vi "编码输出.vi"(8 "error in (no error)":errorcluster, 11 "SingleStepTestV3输入":refnum<class "SingleStepCODMnV2.lvclass">) -> (0 "error out":errorcluster)   [LabVIEW 2016, in "SingleStepCODMnV2.lvlib" / "SingleStepCODMnV2.lvclass"]
uses:
  SingleStepCODMnV2.lvclass
  SingleStepCODMnV2.lvclass/SingleStepCODMnV2.ctl
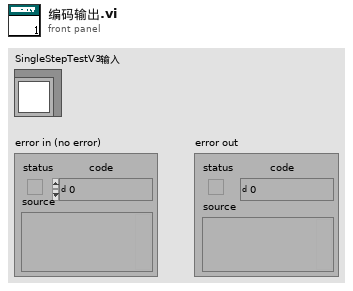
[diagram p1: front panel]
types:
  T1 = enum32{"未选择", "水样", "纯水", "标液", "零点", "加标回收", "加标回收 2"}
  T2 = enum32{"未选择", "纯水-进", "纯水-排", "硫酸-进", "硫酸-排", "复位", "高锰酸钾-进", "高锰酸钾-排", "草酸钠-进", "草酸钠-排", "氢氧化钠-进", "氢氧化钠-排", "反滴定"}
  T3 = enum32{"未选择", "V1", "V2", "V3", "V4", "V5", "V6", "V7", "V8", "V9", "V10", "V11", "V12"}
  T4 = typedef "SingleStepCODMnV2.lvlib/SingleStepCODMnV2.lvclass/State Data.ctl" = cluster{"data":u16[], "模式选择":enum16{"测试模式", "流程模式"}}
  T5 = enum32{"未选择", "水样", "纯水", "标液", "零点", "加标回收", "跨度"}
  T6 = cluster{"排液":bool, "搅拌":bool, "风扇":bool, "废液分离":bool}
  T7 = cluster{"排液阀":bool, "搅拌":bool, "冷凝风扇":bool, "废液分离阀":bool, "电磁阀1":bool, "电磁阀2":bool, "电磁阀3":bool, "电磁阀4":bool, "电磁阀5":bool, "电磁阀6":bool, "电磁阀7":bool}
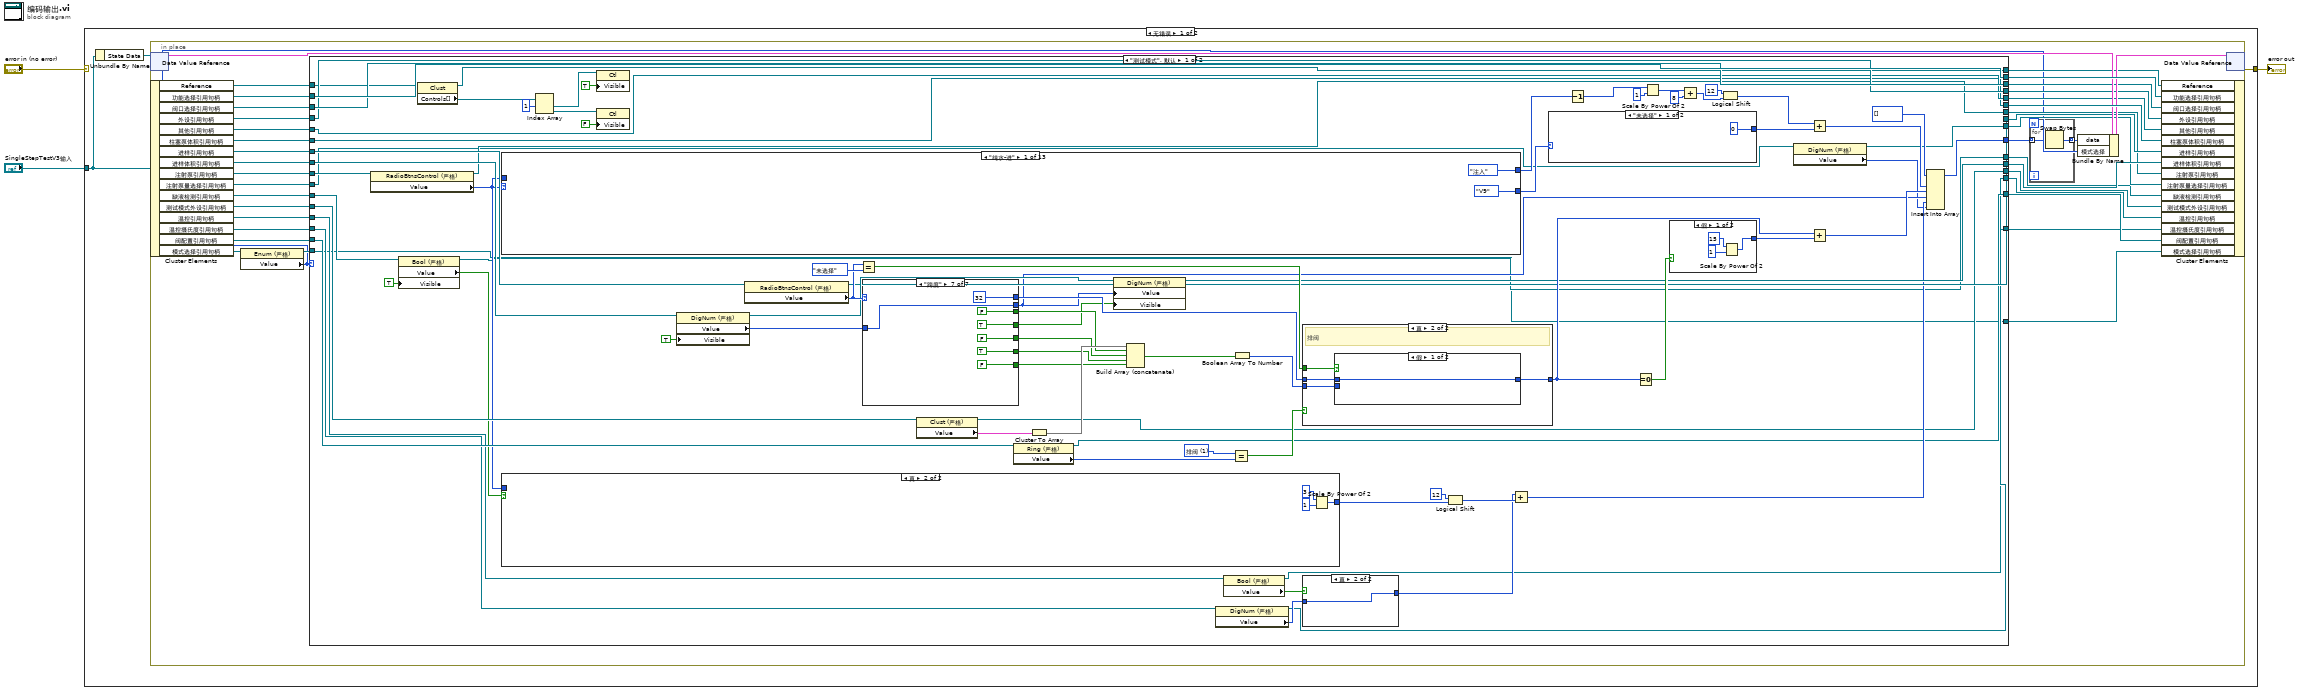
[diagram p0: block diagram]
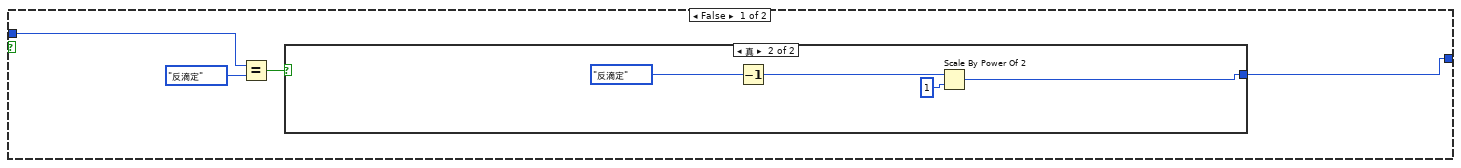
[diagram p2: hidden frame]
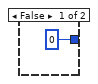
[diagram p3: hidden frame]
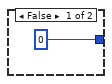
[diagram p4: hidden frame]
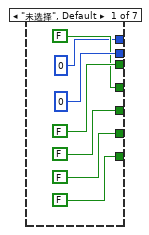
[diagram p5: hidden frame]
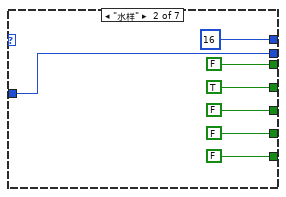
[diagram p6: hidden frame]
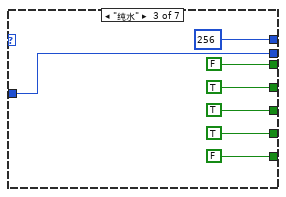
[diagram p7: hidden frame]
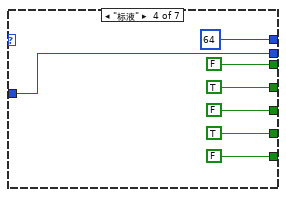
[diagram p8: hidden frame]
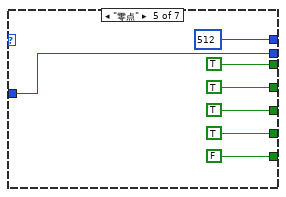
[diagram p9: hidden frame]
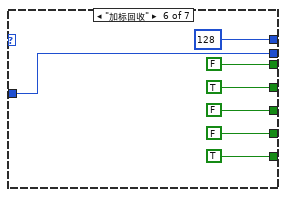
[diagram p10: hidden frame]
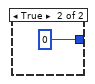
[diagram p13: hidden frame]
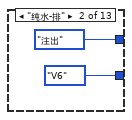
[diagram p14: hidden frame]
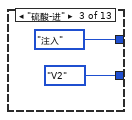
[diagram p15: hidden frame]
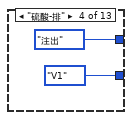
[diagram p16: hidden frame]
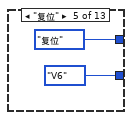
[diagram p17: hidden frame]
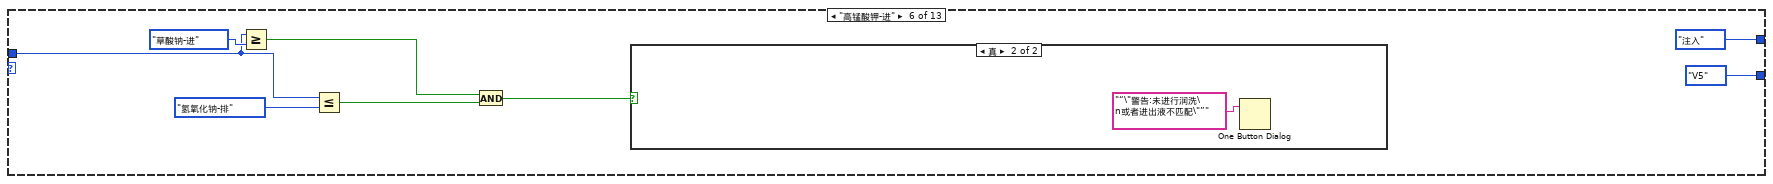
[diagram p18: hidden frame]
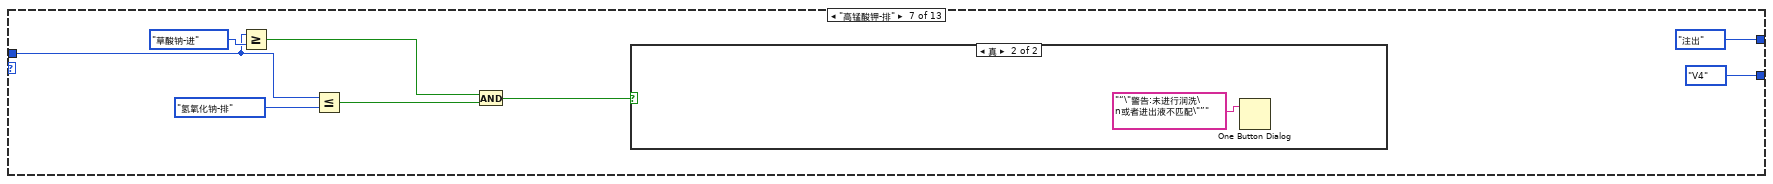
[diagram p20: hidden frame]
diagram:
  n1 = case shown="无错误" "error in (no error)" {
    selector: "error in (no error)" -> [_ w360]
    tunnel: "SingleStepTestV3输入" -> [w5 _]
    tunnel: [w4 w360] -> w2
    frame No Error {
      n2 = Unbundle By Name(w5) -> ("State Data"=w6:refnum<data-value>)
      n3 = in-place {
        n4 = in-place-dvr #1(w6) -> (w40:T4)  [unwired: 1 out]
        n5 = in-place-cluster #2(w5) -> ("Reference"=w9:refnum<vi>, "功能选择引用句柄"=w44:refnum<vi>, "阀口选择引用句柄"=w38:refnum<vi>, "外设引用句柄"=w36:refnum<vi>, "其他引用句柄"=w33:refnum<vi>, "柱塞泵体积引用句柄"=w31:refnum<vi>, "进样引用句柄"=w30:refnum<vi>, "进样体积引用句柄"=w29:refnum<vi>, "注射泵引用句柄"=w28:refnum<vi>, "注射泵量选择引用句柄"=w21:refnum<vi>, "缺液检测引用句柄"=w20:refnum<vi>, "测试模式外设引用句柄"=w26:refnum<vi>, "温控引用句柄"=w22:refnum<vi>, "温控摄氏度引用句柄"=w19:refnum<vi>, "阀配置引用句柄"=w27:refnum<vi>, "模式选择引用句柄"=w11:refnum<vi>)
        n6 = property class="Enum (严格)"(reference=w11) -> (reference out=w10:refnum<vi>, "Value"=w7:enum16{"测试模式", "流程模式"})  [unwired: 1 in, 1 out]
        n7 = case shown="\"测试模式\", 默认" w7 {
          tunnel: w44 -> [w124 w336]
          tunnel: [w124 w335] -> w43
          tunnel: [w120 w334] -> w42
          tunnel: w38 -> [w123 w325]
          tunnel: [w123 w321] -> w37
          tunnel: w36 -> [w122 w320]
          tunnel: [w122 w318] -> w35
          tunnel: [w118 w316] -> w34
          tunnel: w33 -> [w121 w314]
          tunnel: [w121 w307] -> w32
          tunnel: w31 -> [w120 w306]
          tunnel: w30 -> [w105 w301]
          tunnel: w29 -> [w104 w303]
          tunnel: w28 -> [w103 w299]
          tunnel: w27 -> [w97 w293]
          tunnel: w26 -> [w90 w296]
          tunnel: [w79 w301] -> w25
          tunnel: [w78 w300] -> w24
          tunnel: [w77 w299] -> w23
          tunnel: w22 -> [w70 w295]
          tunnel: w21 -> [w68 w298]
          tunnel: w20 -> [w67 w304]
          tunnel: w19 -> [w63 w294]
          tunnel: [w61 w293] -> w18
          tunnel: [w60 w294] -> w17
          tunnel: [w59 w295] -> w16
          tunnel: [w58 w296] -> w15
          tunnel: [w57 w298] -> w14
          tunnel: [w56 w297] -> w13
          tunnel: w10 -> [w54 w292]
          tunnel: [w54 w292] -> w12
          tunnel: w9 -> [w53 w291]
          tunnel: [w46 w284] -> w8
          frame "测试模式", Default {
            w98 = u8 1 items=["三通阀", "排阀"] ("Value")
            n8 = property class="RadioBtnsControl (严格)"(reference=w103) -> (reference out=w77:refnum<vi>, "Value"=w65:T2)  [unwired: 1 in, 1 out]
            n9 = property class="Bool (严格)"(reference=w67, "Visible"=TRUE ("可见")) -> (reference out=w56:refnum<vi>, "Value"=w66:bool)  [unwired: 1 in, 1 out]
            n10 = property class="Clust"(reference=w53) -> (reference out=w46:refnum<vi>, "Controls[]"=w52:refnum<vi>[])  [unwired: 1 in, 1 out]
            n11 = case shown="\"纯水-进\"" w65 {
              tunnel: [enum32{"等待", "复位", "注入", "注出"}."注入" ("功能选择") enum32{"等待", "复位", "注入", "注出"}."注出" ("功能选择") enum32{"等待", "复位", "注入", "注出"}."注入" ("功能选择") enum32{"等待", "复位", "注入", "注出"}."注出" ("功能选择") enum32{"等待", "复位", "注入", "注出"}."复位" ("功能选择") enum32{"等待", "复位", "注入", "注出"}."注入" ("功能选择") enum32{"等待", "复位", "注入", "注出"}."注出" ("功能选择") enum32{"等待", "复位", "注入", "注出"}."注入" ("功能选择") enum32{"等待", "复位", "注入", "注出"}."注出" ("功能选择") enum32{"等待", "复位", "注入", "注出"}."注入" ("功能选择") enum32{"等待", "复位", "注入", "注出"}."注出" ("功能选择") 0 0] -> w108
              tunnel: [T3."V9" ("阀口选择") T3."V6" ("阀口选择") T3."V2" ("阀口选择") T3."V1" ("阀口选择") T3."V6" ("阀口选择") T3."V5" ("阀口选择") T3."V4" ("阀口选择") T3."V7" ("阀口选择") T3."V8" ("阀口选择") T3."V3" ("阀口选择") T3."V6" ("阀口选择") T3."未选择" ("阀口选择") T3."未选择" ("阀口选择")] -> w107
              tunnel: w65 -> [_ _ _ _ _ w209 w218 w227 w242 w257 w266 _ _]
              frame "纯水-进" {
              }
              frame "纯水-排" {
              }
              frame "硫酸-进" {
              }
              frame "硫酸-排" {
              }
              frame "复位" {
              }
              frame "高锰酸钾-进" {
                n12 = Greater Or Equal?(x=w209, y=T2."草酸钠-进" ("注射泵:")) -> (x >= y?=w212:bool)
                n13 = Less Or Equal?(x=w209, y=T2."氢氧化钠-排" ("注射泵:")) -> (x <= y?=w213:bool)
                n14 = And(x=w212, y=w213) -> (x .and. y?=w214:bool)
                n15 = case shown="真" w214 {
                  frame False {
                  }
                  frame True {
                    n16 = One Button Dialog(message="“\"警告:未进行润洗\n或者进出液不匹配\"”" ("消息")) -> ()  [unwired: 1 in, 1 out]
                  }
                }
              }
              frame "高锰酸钾-排" {
                n17 = Greater Or Equal?(x=w218, y=T2."草酸钠-进" ("注射泵:")) -> (x >= y?=w221:bool)
                n18 = Less Or Equal?(x=w218, y=T2."氢氧化钠-排" ("注射泵:")) -> (x <= y?=w222:bool)
                n19 = And(x=w221, y=w222) -> (x .and. y?=w223:bool)
                n20 = case shown="真" w223 {
                  frame False {
                  }
                  frame True {
                    n21 = One Button Dialog(message="“\"警告:未进行润洗\n或者进出液不匹配\"”" ("消息")) -> ()  [unwired: 1 in, 1 out]
                  }
                }
              }
              frame "草酸钠-进" {
                n22 = Greater Or Equal?(x=w227, y=T2."氢氧化钠-进" ("注射泵:")) -> (x >= y?=w230:bool)
                n23 = Less Or Equal?(x=w227, y=T2."氢氧化钠-排" ("注射泵:")) -> (x <= y?=w229:bool)
                n24 = Greater Or Equal?(x=w227, y=T2."高锰酸钾-进" ("注射泵:")) -> (x >= y?=w235:bool)
                n25 = Less Or Equal?(x=w227, y=T2."高锰酸钾-排" ("注射泵:")) -> (x <= y?=w236:bool)
                n26 = And(x=w230, y=w229) -> (x .and. y?=w228:bool)
                n27 = And(x=w235, y=w236) -> (x .and. y?=w237:bool)
                n28 = Or(x=w228, y=w237) -> (x .or. y?=w238:bool)
                n29 = case shown="真" w238 {
                  frame False {
                  }
                  frame True {
                    n30 = One Button Dialog(message="“\"警告:未进行润洗\n或者进出液不匹配\"”" ("消息")) -> ()  [unwired: 1 in, 1 out]
                  }
                }
              }
              frame "草酸钠-排" {
                n31 = Less Or Equal?(x=w242, y=T2."氢氧化钠-排" ("注射泵:")) -> (x <= y?=w244:bool)
                n32 = Greater Or Equal?(x=w242, y=T2."高锰酸钾-进" ("注射泵:")) -> (x >= y?=w250:bool)
                n33 = Greater Or Equal?(x=w242, y=T2."氢氧化钠-进" ("注射泵:")) -> (x >= y?=w245:bool)
                n34 = Less Or Equal?(x=w242, y=T2."高锰酸钾-排" ("注射泵:")) -> (x <= y?=w251:bool)
                n35 = And(x=w245, y=w244) -> (x .and. y?=w243:bool)
                n36 = And(x=w250, y=w251) -> (x .and. y?=w252:bool)
                n37 = Or(x=w243, y=w252) -> (x .or. y?=w253:bool)
                n38 = case shown="真" w253 {
                  frame False {
                  }
                  frame True {
                    n39 = One Button Dialog(message="“\"警告:未进行润洗\n或者进出液不匹配\"”" ("消息")) -> ()  [unwired: 1 in, 1 out]
                  }
                }
              }
              frame "氢氧化钠-进" {
                n40 = Less Or Equal?(x=w257, y=T2."草酸钠-排" ("注射泵:")) -> (x <= y?=w262:bool)
                n41 = Greater Or Equal?(x=w257, y=T2."高锰酸钾-进" ("注射泵:")) -> (x >= y?=w261:bool)
                n42 = And(x=w261, y=w262) -> (x .and. y?=w258:bool)
                n43 = case shown="真" w258 {
                  frame False {
                  }
                  frame True {
                    n44 = One Button Dialog(message="“\"警告:未进行润洗\n或者进出液不匹配\"”" ("消息")) -> ()  [unwired: 1 in, 1 out]
                  }
                }
              }
              frame "氢氧化钠-排" {
                n45 = Less Or Equal?(x=w266, y=T2."草酸钠-排" ("注射泵:")) -> (x <= y?=w271:bool)
                n46 = Greater Or Equal?(x=w266, y=T2."高锰酸钾-进" ("注射泵:")) -> (x >= y?=w270:bool)
                n47 = And(x=w270, y=w271) -> (x .and. y?=w267:bool)
                n48 = case shown="真" w267 {
                  frame False {
                  }
                  frame True {
                    n49 = One Button Dialog(message="“\"警告:未进行润洗\n或者进出液不匹配\"”" ("消息")) -> ()  [unwired: 1 in, 1 out]
                  }
                }
              }
              frame "反滴定" {
              }
              frame "未选择" {
              }
            }
            n50 = case shown="真" w66 {
              tunnel: w65 -> [w127 _]
              tunnel: [w125 w135] -> w72
              frame False {
                n51 = Equal?(x=w127, y=T2."反滴定" ("注射泵:")) -> (x = y?=w126:bool)
                n52 = case shown="真" w126 {
                  tunnel: [i16 0 w130] -> w125
                  frame False {
                  }
                  frame True {
                    n53 = Decrement(x=enum32{"未选择", "更新A值", "更新B值", "反滴定"}."反滴定" ("其他")) -> (x-1=w131:enum32{"未选择", "更新A值", "更新B值", "反滴定"})
                    n54 = Scale By Power Of 2(n=w131, x=i16 1 ("y")) -> (x*2^n=w130:i16)
                  }
                }
              }
              frame True {
                n55 = Scale By Power Of 2(n=i16 3, x=i16 1 ("y")) -> (x*2^n=w135:i16)
              }
            }
            n56 = Index Array(array=w52, index #1=1 ("索引")) -> (element #1=w50:refnum<vi>, element #2=w49:refnum<vi>)  [unwired: 1 in]
            n57 = property class="Ctl"(reference=w50, "Visible"=TRUE ("可见")) -> ()  [unwired: 1 in, 2 out]
            n58 = property class="Ctl"(reference=w49, "Visible"=FALSE ("可见")) -> ()  [unwired: 1 in, 2 out]
            n59 = property class="DigNum (严格)"(reference=w104, "Visible"=TRUE ("可见")) -> (reference out=w81:refnum<vi>, "Value"=w92:u16)  [unwired: 1 in, 1 out]
            n60 = property class="RadioBtnsControl (严格)"(reference=w105) -> (reference out=w79:refnum<vi>, "Value"=w93:T5)  [unwired: 1 in, 1 out]
            n61 = Equal?(x=w93, y=T1."未选择") -> (x = y?=w94:bool)
            n62 = case shown="\"跨度\"" w93 {
              tunnel: [FALSE FALSE FALSE FALSE TRUE FALSE FALSE] -> w85
              tunnel: [FALSE FALSE TRUE FALSE TRUE FALSE FALSE] -> w84
              tunnel: [FALSE FALSE TRUE TRUE TRUE FALSE TRUE] -> w83
              tunnel: [FALSE FALSE FALSE FALSE FALSE TRUE FALSE] -> w82
              tunnel: w92 -> [_ w148 w155 w162 w169 w176 w186]
              tunnel: [u16 0 ("偏心轮:") w148 w155 w162 w169 w176 w186] -> w76
              tunnel: [FALSE TRUE TRUE TRUE TRUE TRUE TRUE] -> w80
              tunnel: [u16 0 ("数字") u16 16 ("数字") u16 256 ("数字") u16 64 ("数字") u16 512 ("数字") u16 128 ("数字") u16 32 ("数字")] -> w91
              frame "未选择", Default {
              }
              frame "水样" {
              }
              frame "纯水" {
              }
              frame "标液" {
              }
              frame "零点" {
              }
              frame "加标回收" {
              }
              frame "跨度" {
              }
            }
            n63 = property class="Clust (严格)"(reference=w90) -> (reference out=w58:refnum<vi>, "Value"=w89:T6)  [unwired: 1 in, 1 out]
            n64 = property class="Ring (严格)"(reference=w97) -> (reference out=w61:refnum<vi>, "Value"=w96:u8)  [unwired: 1 in, 1 out]
            n65 = Cluster To Array(cluster=w89) -> (array=w86:bool[])
            n66 = property class="DigNum (严格)"(reference=w81, "Value"=w76, "Visible"=w80) -> (reference out=w78:refnum<vi>)  [unwired: 1 in, 1 out]
            n67 = Build Array (concatenate)(w86, w85, w84, w83, w82) -> (w88:bool[])
            n68 = property class="DigNum (严格)"(reference=w63) -> (reference out=w60:refnum<vi>, "Value"=w62:u16)  [unwired: 1 in, 1 out]
            n69 = property class="Bool (严格)"(reference=w70) -> (reference out=w59:refnum<vi>, "Value"=w69:bool)  [unwired: 1 in, 1 out]
            n70 = Equal?(x=w98, y=w96) -> (x = y?=w95:bool)
            n71 = Boolean Array To Number ("布尔数组至数值转换")(Boolean array=w88) -> (number=w87:u16)
            n72 = case shown="真" w95 {
              tunnel: w87 -> [w188 w192]
              tunnel: [w188 w191] -> w99
              tunnel: w91 -> [_ w190]
              tunnel: w94 -> [_ w189]
              frame False {
              }
              frame True {
                # "排阀"
                n73 = case shown="假" w189 {
                  tunnel: w192 -> [_ w194]
                  tunnel: [w193 w194] -> w191
                  tunnel: w190 -> [w193 _]
                  frame False {
                  }
                  frame True {
                  }
                }
              }
            }
            n74 = case shown="真" w69 {
              tunnel: [u16 0 ("摄氏度") w138] -> w73
              tunnel: w62 -> [_ w138]
              frame False {
              }
              frame True {
              }
            }
            n75 = Logical Shift(y=i16 12, x=w72) -> (x << y=w74:i16)
            n76 = Add(x=w73, y=w74) -> (x+y=w71:u16)
            n77 = case shown="\"未选择\"" w107 {
              selector: w107 -> [_ w281]
              tunnel: [i16 0 ("y") w283] -> w117
              frame "未选择" {
              }
              frame Default {
                n78 = Decrement(x=w281) -> (x-1=w282:T3)
                n79 = Scale By Power Of 2(n=w282, x=i16 1 ("y")) -> (x*2^n=w283:i16)
              }
            }
            n80 = Decrement(x=w108) -> (x-1=w110:u32)
            n81 = Equal To 0?(x=w99) -> (x = 0?=w101:bool)
            n82 = Scale By Power Of 2(n=w110, x=i16 1 ("y")) -> (x*2^n=w113:i16)
            n83 = case shown="假" w101 {
              tunnel: [w195 u16 0] -> w102
              frame False {
                n84 = Scale By Power Of 2(n=i16 15, x=u16 1 ("y")) -> (x*2^n=w195:u16)
              }
              frame True {
              }
            }
            n85 = Add(x=w113, y=i16 8) -> (x+y=w114:i16)
            n86 = Logical Shift(y=i16 12, x=w114) -> (x << y=w116:i16)
            n87 = property class="DigNum (严格)"(reference=w68) -> (reference out=w57:refnum<vi>, "Value"=w64:u16)  [unwired: 1 in, 1 out]
            n88 = Add(x=w116, y=w117) -> (x+y=w109:i16)
            n89 = Add(x=w99, y=w102) -> (x+y=w100:u16)
            n90 = Insert Into Array(array=u16[] [] ("数组"), new element #1=w109, new element #2=w100, new element #3=w76, new element #4=w71, new element #5=w64) -> (w118:u16[])  [unwired: 1 in]
          }
          frame "流程模式" {
            w302 = FALSE
            w309 = u16 0  # 反应杯温度控制
            w315 = u16 0  # 偏心轮次数
            n91 = property class="Clust"(reference=w291) -> (reference out=w284:refnum<vi>, "Controls[]"=w290:refnum<vi>[])  [unwired: 1 in, 1 out]
            n92 = property class="DigNum (严格)"(reference=w303, "Visible"=w302) -> (reference out=w300:refnum<vi>)  [unwired: 1 in, 1 out]
            n93 = property class="Bool (严格)"(reference=w304, "Visible"=w302) -> (reference out=w297:refnum<vi>)  [unwired: 1 in, 1 out]
            n94 = Index Array(array=w290, index #1=1 ("索引")) -> (element #1=w288:refnum<vi>, element #2=w287:refnum<vi>)  [unwired: 1 in]
            n95 = property class="Ctl"(reference=w288, "Visible"=FALSE) -> ()  [unwired: 1 in, 2 out]
            n96 = property class="Ctl"(reference=w287, "Visible"=TRUE) -> ()  [unwired: 1 in, 2 out]
            n97 = property class="RadioBtnsControl (严格)"(reference=w336) -> (reference out=w335:refnum<vi>, "Value"=w333:enum32{"等待", "复位", "注入", "注出"})  [unwired: 1 in, 1 out]
            n98 = case shown="\"复位\", 默认" w333 {
              selector: w333 -> [_ w350]
              tunnel: [u16 1 ("y") u16 0 ("y")] -> w326
              tunnel: [i16 0 ("y") w349] -> w327
              frame "等待" {
              }
              frame "复位", Default {
                n99 = Decrement(x=w350) -> (x-1=w351:enum32{"等待", "复位", "注入", "注出"})
                n100 = Scale By Power Of 2(n=w351, x=i16 1 ("y")) -> (x*2^n=w354:i16)
                n101 = Add(x=w354, y=i16 8) -> (x+y=w353:i16)
                n102 = Logical Shift(y=i16 12, x=w353) -> (x << y=w349:i16)
              }
            }
            n103 = property class="RadioBtnsControl (严格)"(reference=w325) -> (reference out=w321:refnum<vi>, "Value"=w324:T3)  [unwired: 1 in, 1 out]
            n104 = case shown="默认" w324 {
              selector: w324 -> [_ w344]
              tunnel: [i16 0 ("y") w346] -> w323
              frame "未选择" {
              }
              frame Default {
                n105 = Decrement(x=w344) -> (x-1=w345:T3)
                n106 = Scale By Power Of 2(n=w345, x=i16 1 ("y")) -> (x*2^n=w346:i16)
              }
            }
            n107 = property class="RadioBtnsControl (严格)"(reference=w314) -> (reference out=w307:refnum<vi>, "Value"=w313:enum32{"未选择", "更新A值", "更新B值", "反滴定"})  [unwired: 1 in, 1 out]
            n108 = case shown="\"未选择\"" w313 {
              selector: w313 -> [_ w338]
              tunnel: [i16 0 w339] -> w311
              frame "未选择" {
              }
              frame "更新A值", Default {
                n109 = Decrement(x=w338) -> (x-1=w341:enum32{"未选择", "更新A值", "更新B值", "反滴定"})
                n110 = Scale By Power Of 2(n=w341, x=i16 1 ("y")) -> (x*2^n=w339:i16)
              }
            }
            n111 = property class="Clust (严格)"(reference=w320) -> (reference out=w318:refnum<vi>, "Value"=w319:T7)  [unwired: 1 in, 1 out]
            n112 = Cluster To Array(cluster=w319) -> (array=w329:bool[])
            n113 = Add(x=w327, y=w323) -> (x+y=w322:i16)
            n114 = Boolean Array To Number ("布尔数组至数值转换")(Boolean array=w329) -> (number=w330:u16)
            n115 = Scale By Power Of 2(n=i16 15, x=w326) -> (x*2^n=w331:u16)
            n116 = Logical Shift(y=i16 12, x=w311) -> (x << y=w310:i16)
            n117 = property class="DigNum (严格)"(reference=w306) -> (reference out=w334:refnum<vi>, "Value"=w305:u16)  [unwired: 1 in, 1 out]
            n118 = Add(x=w330, y=w331) -> (x+y=w317:u16)
            n119 = Add(x=w309, y=w310) -> (x+y=w308:u16)
            n120 = Insert Into Array(array=u16[] [] ("数组"), new element #1=w322, new element #2=w317, new element #3=w315, new element #4=w308, new element #5=w305) -> (w316:u16[])  [unwired: 1 in]
          }
        }
        n121 = for {
          tunnel: [w359] -> w39 mode=indexing
          tunnel: w34 -> [w358] mode=indexing
          n122 = Swap Bytes(anything=w358) -> (byte swapped=w359:u16)
        }
        n123 = Bundle By Name(cluster=w40, "data"=w39, "模式选择"=w7) -> (w41:T4)
        n124 = in-place-cluster #2("Reference"=w8, "功能选择引用句柄"=w43, "阀口选择引用句柄"=w37, "外设引用句柄"=w35, "其他引用句柄"=w32, "柱塞泵体积引用句柄"=w42, "进样引用句柄"=w25, "进样体积引用句柄"=w24, "注射泵引用句柄"=w23, "注射泵量选择引用句柄"=w14, "缺液检测引用句柄"=w13, "测试模式外设引用句柄"=w15, "温控引用句柄"=w16, "温控摄氏度引用句柄"=w17, "阀配置引用句柄"=w18, "模式选择引用句柄"=w12) -> ()  [unwired: 1 out]
        n125 = in-place-dvr #1(w41) -> (w4:errorcluster)  [unwired: 1 out]
      }
    }
    frame Error {
    }
  }
  "error out" <- w2
